vi "toString.vi"(8 "error in (no error)":errorcluster, 11 "Status in":refnum<class "Status.lvclass">) -> (0 "error out":errorcluster, 2 "String":string, 3 "Status out":refnum<class "Status.lvclass">)   [LabVIEW 2017, in "Message Interface.lvlib" / "Status.lvclass"]
uses:
  Status.lvclass
  Status.lvclass/Status.ctl
  iMessage/iMessage.lvclass
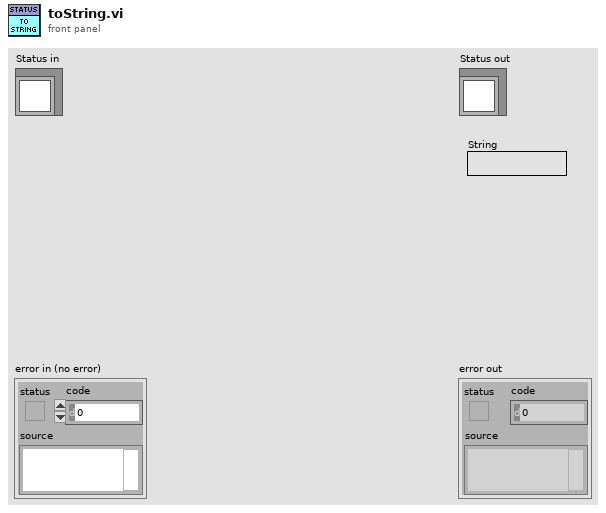
[diagram p1: front panel]
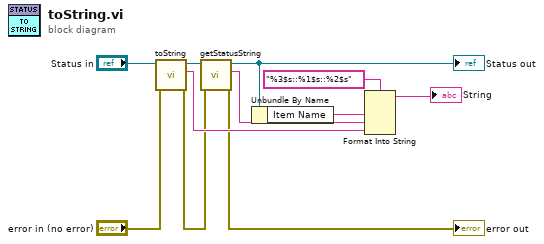
[diagram p0: block diagram]
diagram:
  n1 = call-parent "toString.vi"("error in (no error)"="error in (no error)", "iMessage in"="Status in") -> ("error out"=w2:errorcluster, "String"=w8:string, "iMessage out"=w5:refnum<class "Status.lvclass">)  [unwired: 7 in]
  n2 = call-dynamic "getStatusString.vi"("error in (no error)"=w2, "Status in"=w5) -> ("error out"=→"error out":errorcluster, "Status String"=w3:string, "Status out"=w4:refnum<class "Status.lvclass">)  [unwired: 7 in]
  "Status out" <- w4
  n3 = Unbundle By Name(w4) -> ("Item Name"=w9:string)
  n4 = Format Into String(format string="%3$s::%1$s::%2$s", w9, w3, w8) -> (resulting string=→"String":string)  [unwired: 2 in, 1 out]
